vi "String Functions 2b.vi"() -> ()   [LabVIEW 2020]
panel:
  out "Data":string="Data"
  out "Command":string="Command"
  in  "Message From Hardware":string="Command | Data"
  # "Simulate a message from a hardware device by typing a string in this format:\n<Command> | <Data>"
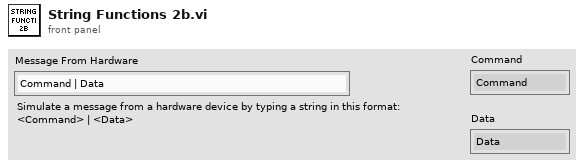
[diagram p1: front panel]
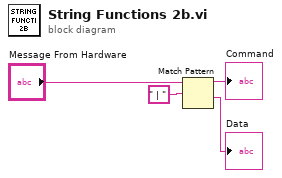
[diagram p0: block diagram]
diagram:
  n1 = Match Pattern(string="Message From Hardware", regular expression=" | ") -> (before substring=→"Command":string, after substring=→"Data":string)  [unwired: 1 in, 2 out]
